vi "NegativeTimeString.vi"(1 "Time(s)":dbl) -> (0 "Relative time string":string)   [LabVIEW 2015]
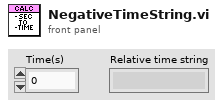
[diagram p1: front panel]
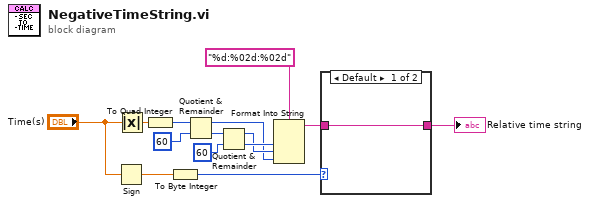
[diagram p0: block diagram]
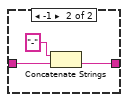
[diagram p2: hidden frame]
diagram:
  n1 = Sign(1:"Time(s)") -> (0:w13:dbl)
  n2 = Absolute Value(x="Time(s)") -> (abs(x)=w10:dbl)
  n3 = To Quad Integer(1:w10) -> (0:w9:i64)
  n4 = To Byte Integer(number=w13) -> (8bit integer=w12:i8)
  n5 = Quotient & Remainder(x=w9, y=i64 60) -> (x-y*floor(x/y)=w2:i64, floor(x/y)=w7:i64)
  n6 = Quotient & Remainder(x=w7, y=i64 60) -> (x-y*floor(x/y)=w3:i64, floor(x/y)=w4:i64)
  n7 = Format Into String(format string="%d:%02d:%02d", w4, w3, w2) -> (resulting string=w1:string)  [unwired: 2 in, 1 out]
  n8 = case shown="Default" w12 {
    tunnel: [w15 w16] -> w11
    tunnel: w1 -> [w15 w18]
    frame Default {
    }
    frame -1 {
      n9 = Concatenate Strings("-" ("string"), w18) -> (w16:string)
    }
  }
  "Relative time string" <- w11
